vi "CliIsoExchangeBuffer.vi"(0 "ref in":u64, 7 "data in":string, 9 "Size in":i32, 11 "error in (no error)":errorcluster) -> (4 "ref out":u64, 6 "Result":i32, 8 "data out":string, 10 "Size out":i32, 15 "error out":errorcluster)   [LabVIEW 2019, in "Snap7.lvlib"]
uses:
  Snap7.lvlib
  windows/lv_snap7.dll
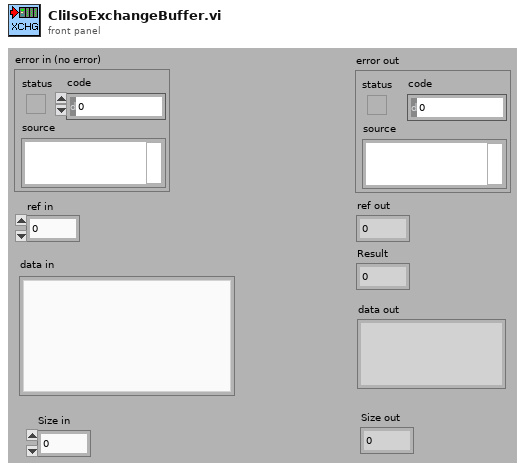
[diagram p1: front panel]
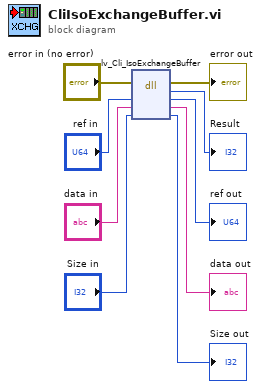
[diagram p0: block diagram]
diagram:
  n1 = dll-call lib="PTH2Xabs DSVNHLCEPStrunk性能试验台SourcesSnap7libwindowslv_snap7.dll" fn="lv_Cli_IsoExchangeBuffer"(error in="error in (no error)", "Client"="ref in", "pUsrData"="data in", "Size"="Size in") -> (error out=→"error out":errorcluster, "return type"=→"Result":i32, "Client"=→"ref out":u64, "pUsrData"=→"data out":string, "Size"=→"Size out":i32)  [unwired: 2 in, 1 out]
